vi "2.2.vi"() -> ()   [LabVIEW 2017]
panel:
  out "x*y":i32
  out "dist":i32
  out "depth":i32
  in  "String":string
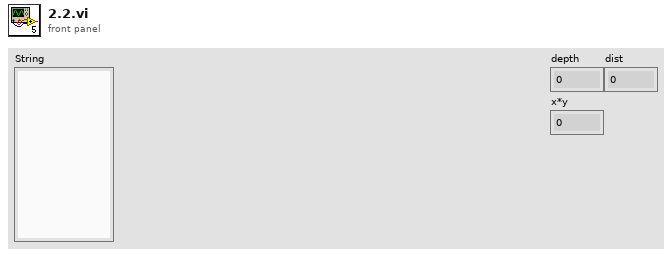
[diagram p1: front panel]
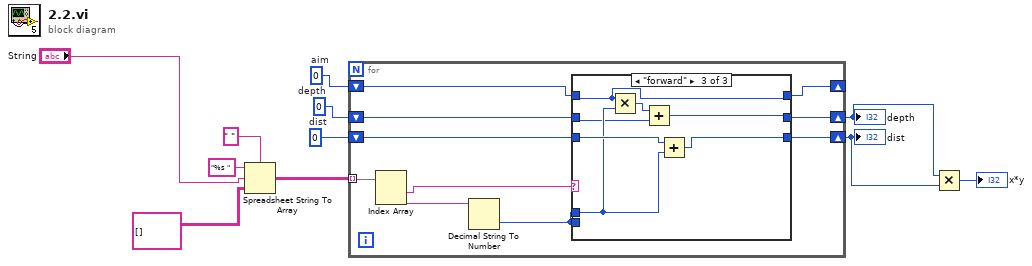
[diagram p0: block diagram]
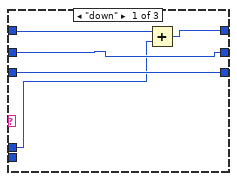
[diagram p2: hidden frame]
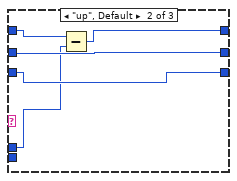
[diagram p3: hidden frame]
diagram:
  w1 = 0  # aim
  w6 = 0  # dist
  w5 = 0  # depth
  n1 = Spreadsheet String To Array(delimiter (Tab)=" ", format string="%s ", spreadsheet string="String", array type (2D Dbl)=string[][] []) -> (array=w7:string[][])
  n2 = for {
    tunnel: w7 -> [w21] mode=indexing
    shift-right: [w16] -> w4
    shift-left: w5 -> [w17]
    shift-right: [w15] -> w3
    shift-left: w6 -> [w18]
    shift-right: [w13] -> _
    shift-left: w1 -> [w12]
    n3 = Index Array(array=w21) -> (element #1=w19:string, element #2=w20:string)  [unwired: 2 in]
    n4 = Decimal String To Number(string=w20) -> (number=w14:i32)  [unwired: 2 in, 1 out]
    n5 = case shown="\"forward\"" w19 {
      tunnel: w18 -> [w26 w31 w38]
      tunnel: w17 -> [w25 w30 w34]
      tunnel: [w25 w30 w33] -> w16
      tunnel: [w26 w31 w37] -> w15
      tunnel: w14 -> [_ _ _]
      tunnel: w14 -> [w23 w28 w36]
      tunnel: [w22 w27 w32] -> w13
      tunnel: w12 -> [w24 w29 w32]
      frame "down" {
        n6 = Add(x=w24, y=w23) -> (x+y=w22:i32)
      }
      frame "up", Default {
        n7 = Subtract(x=w29, y=w28) -> (x-y=w27:i32)
      }
      frame "forward" {
        n8 = Multiply(x=w32, y=w36) -> (x*y=w35:i32)
        n9 = Add(x=w35, y=w34) -> (x+y=w33:i32)
        n10 = Add(x=w38, y=w36) -> (x+y=w37:i32)
      }
    }
  }
  "depth" <- w4
  "dist" <- w3
  n11 = Multiply(x=w4, y=w3) -> (x*y=→"x*y":i32)
